vi "Execute Command.vi"(8 "error in (no error)":errorcluster, 10 "UI Populate Menu in":refnum<class "UI Populate Menu.lvclass">, 11 "User Interface References":T1={"This VI"=refnum, "User Interace Plugin"=refnum, "UI Picture Container References"={"Header Image"=refnum, "Footer Image"=refnum}, "Sliding Menu XControl"=refnum, "Menu Container"=refnum, "UI Configuration Information"={"Space Between Buttons"=3, "Number of Buttons to Show"=6, "Header Image"=path "Images/Blue Background.bmp", "Footer Image"=path "Images/Blue Background.bmp"}, "Header Text"=refnum}) -> (0 "error out":errorcluster, 1 "Stop?":bool, 2 "UI Populate Menu out":refnum<class "UI Populate Menu.lvclass">, 3 "User Interface References Out":T1={"This VI"=refnum, "User Interace Plugin"=refnum, "UI Picture Container References"={"Header Image"=refnum, "Footer Image"=refnum}, "Sliding Menu XControl"=refnum, "Menu Container"=refnum, "UI Configuration Information"={"Space Between Buttons"=3, "Number of Buttons to Show"=6, "Header Image"=path "Images/Blue Background.bmp", "Footer Image"=path "Images/Blue Background.bmp"}, "Header Text"=refnum})   [LabVIEW 2011, in "UI Populate Menu.lvclass"]
uses:
  UI Populate Menu.lvclass
  Main Type Definitions/User Interface Type Definitions.ctl
  Sliding Menu/Sliding Menu Library/Sliding Menu SubVIs/Sliding Menu Type Definitions/UI Picture Containers.ctl
  Sliding Menu/Sliding Menu Library/Sliding Menu xControl/Sliding Menu XControl.xctl
  UI Control Definitions/UI Configuration Information.ctl
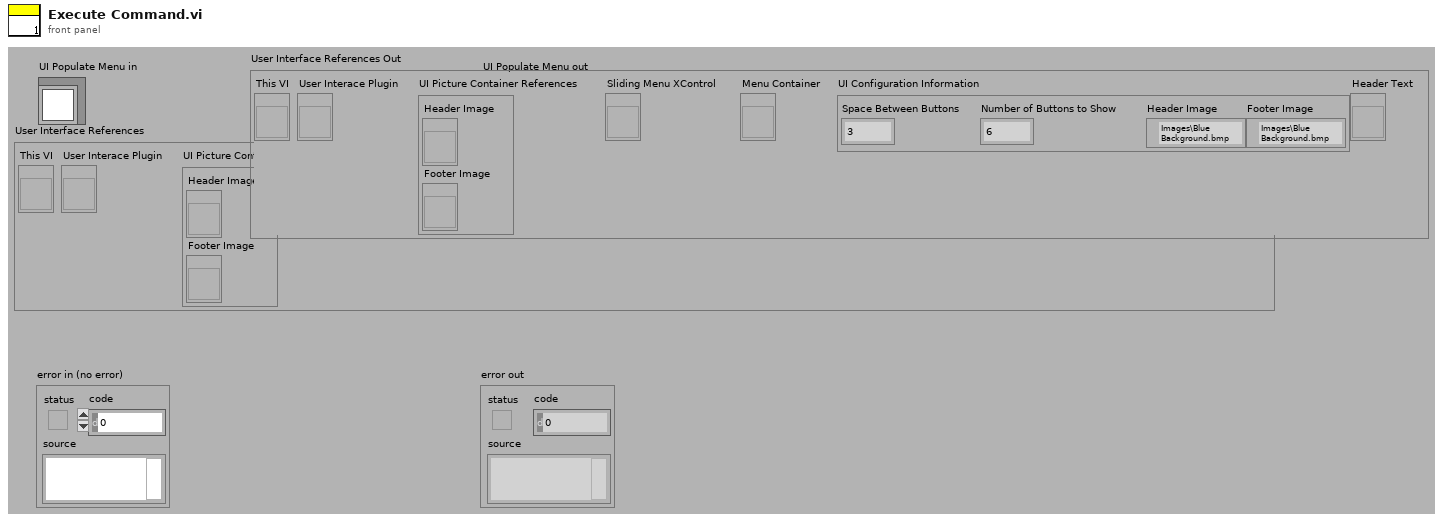
[diagram p1: front panel]
types:
  T1 = typedef "User Interface Type Definitions.ctl" = cluster{"This VI":refnum<vi>, "User Interace Plugin":refnum<vi>, "UI Picture Container References":T2, "Sliding Menu XControl":refnum<vi>, "Menu Container":refnum<vi>, "UI Configuration Information":T3, "Header Text":refnum<vi>}
  T2 = typedef "UI Picture Containers.ctl" = cluster{"Header Image":refnum<vi>, "Footer Image":refnum<vi>}
  T3 = typedef "UI Configuration Information.ctl" = cluster{"Space Between Buttons":i32, "Number of Buttons to Show":i32, "Header Image":path, "Footer Image":path}
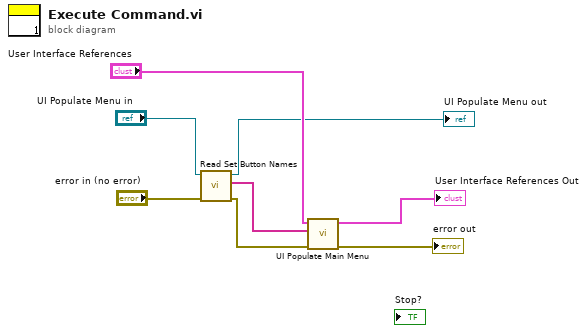
[diagram p0: block diagram]
diagram:
  n1 = call-dynamic "Read Set Button Names.vi"("error in (no error)"="error in (no error)", "UI Populate Menu in"="UI Populate Menu in") -> ("error out"=w3:errorcluster, "Set Button Names"=w6:string[], "UI Populate Menu out"=→"UI Populate Menu out":refnum<class "UI Populate Menu.lvclass">)  [unwired: 7 in]
  n2 = call "UI Populate Main Menu.vi"("error in (no error)"=w3, "Set Button Names"=w6, "User Interface References"="User Interface References") -> ("error out"=→"error out":errorcluster, "User Interface References Out"=→"User Interface References Out":T1)  [unwired: 7 in]
